vi "AxB.vi"(10 "B":dbl[][](array[numeric]), 11 "A":dbl[][](array[numeric])) -> (3 "AxB":T1)   [LabVIEW 2011]
uses:
  <vilib>/Analysis/Matrix/Datatypes/RealMatrix.ctl
  <vilib>/Analysis/Matrix/Numeric/Conversions/Array To Matrix - RA2.vi
  <vilib>/Analysis/Matrix/NI_Matrix.lvlib
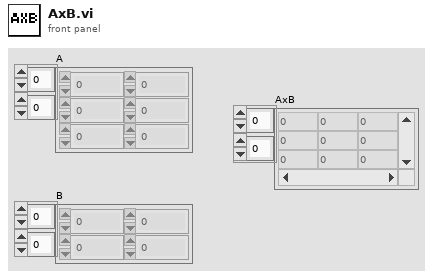
[diagram p1: front panel]
types:
  T1 = typedef "NI_Matrix.lvlib/RealMatrix.ctl" = dbl[][]
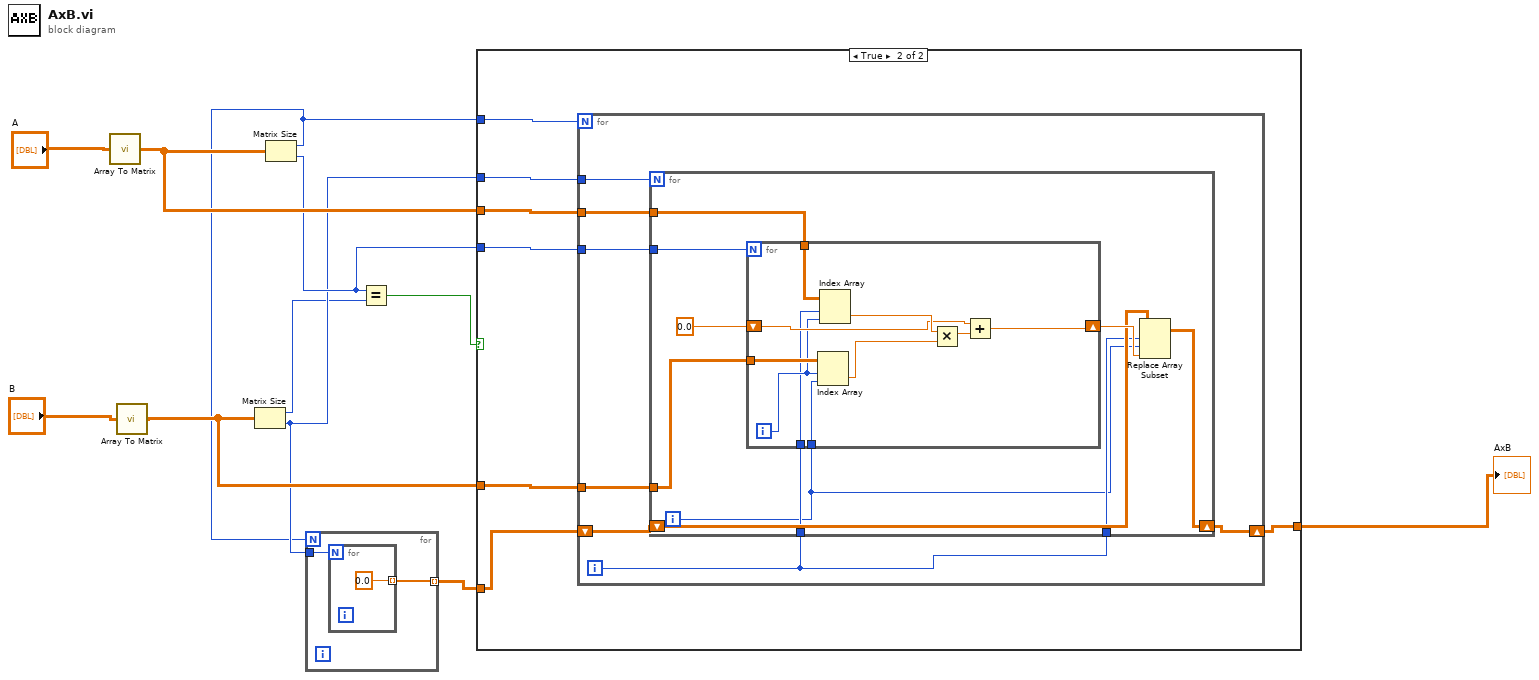
[diagram p0: block diagram]
diagram:
  n1 = call-poly <vilib>:"Array To Matrix.vi"("Real 2D Array"="A") -> ("Real Matrix"=w10:T1)
  n2 = call-poly <vilib>:"Array To Matrix.vi"("Real 2D Array"="B") -> ("Real Matrix"=w9:T1)
  n3 = Matrix Size(0:w9) -> (1:w1:i32, 2:w4:i32)
  n4 = Matrix Size(0:w10) -> (1:w3:i32, 2:w5:i32)
  n5 = for {
    N: w3 -> [_]
    tunnel: [w13] -> w6 mode=indexing
    tunnel: w4 -> [w12]
    n6 = for {
      N: w12 -> [_]
      tunnel: [0.0] -> w13 mode=indexing
    }
  }
  n7 = Equal?(x=w5, y=w1) -> (x = y?=w2:bool)
  n8 = case shown="True" w2 {
    tunnel: w9 -> [_ w21]
    tunnel: w10 -> [_ w20]
    tunnel: w3 -> [_ w19]
    tunnel: w4 -> [_ w18]
    tunnel: w6 -> [_ w17]
    tunnel: w5 -> [_ w16]
    tunnel: [_ w15] -> w7
    frame False {
    }
    frame True {
      n9 = for {
        N: w19 -> [_]
        tunnel: w21 -> [w28]
        tunnel: w20 -> [w27]
        tunnel: w18 -> [w26]
        tunnel: w16 -> [w24]
        shift-right: [w23] -> w15
        shift-left: w17 -> [w25]
        i -> [w22]
        n10 = for {
          N: w26 -> [_]
          tunnel: w28 -> [w35]
          tunnel: w27 -> [w36]
          tunnel: w24 -> [w38]
          shift-right: [w33] -> w23
          shift-left: w25 -> [w32]
          tunnel: w22 -> [w31]
          tunnel: w22 -> [w30]
          i -> [w29]
          n11 = for {
            N: w38 -> [_]
            tunnel: w36 -> [w48]
            tunnel: w35 -> [w47]
            shift-right: [w39] -> w34
            shift-left: 0.0 -> [w44]
            tunnel: w31 -> [w41]
            tunnel: w29 -> [w40]
            i -> [w42]
            n12 = Index Array(array=w47, index (row)=w42, index (col)=w40) -> (element=w45:dbl)
            n13 = Index Array(array=w48, index (row)=w41, index (col)=w42) -> (element=w46:dbl)
            n14 = Multiply(x=w46, y=w45) -> (x*y=w43:dbl)
            n15 = Add(x=w44, y=w43) -> (x+y=w39:dbl)
          }
          n16 = Replace Array Subset(array=w32, new element=w34, index (row)=w30, index (col)=w29) -> (w33:T1)
        }
      }
    }
  }
  "AxB" <- w7
